vi "GlobalYAW.vi"() -> ()   [LabVIEW 2020]
panel:
  out "Yaw":dbl
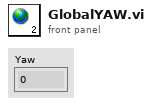
[diagram p1: front panel]
diagram:
